vi "Generate Dashboard DVR.vi"(8 "Error In":errorcluster, 10 "Data":T1, 11 "Dashboard In":refnum<class "Dashboard.lvclass">) -> (0 "Error Out":errorcluster, 3 "Dashboard Out":refnum<class "Dashboard.lvclass">)   [LabVIEW 2019, in "Dashboard.lvclass"]
uses:
  Dashboard.lvclass
  Controls/Data.ctl
  Central Message Handler/Central Message Handler.lvclass
  <vilib>/Memosfet/myRIO-Neopixel/RT/Display/Display.lvclass
  Display Manager/Display Manager.lvclass
  Audio Analyzer/Audio Analyzer.lvclass
  Draw Frame/Draw Frame.lvclass
  Error Handling/Error Handling.lvclass
  Sequencer/Sequencer.lvclass
  <vilib>/Memosfet/OpenWeatherAPI/Open Weather Session/Open Weather Session.lvclass
  Public/Controls/FPGA Reference.ctl
  Controls/Processes.ctl
  Dashboard.lvclass/Dashboard.ctl
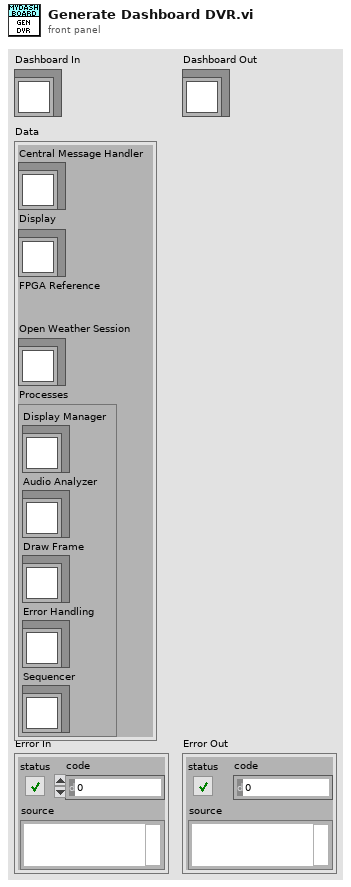
[diagram p1: front panel]
types:
  T1 = typedef "Dashboard.lvclass/Data.ctl" = cluster{"Central Message Handler":refnum<class "Central Message Handler.lvclass">, "Display":refnum<class "Display.lvclass">, "FPGA Reference":T2, "Open Weather Session":refnum<class "Open Weather Session.lvclass">, "Processes":T3}
  T2 = typedef "Dashboard.lvclass/FPGA Reference.ctl" = refnum<k20>
  T3 = typedef "Dashboard.lvclass/Processes.ctl" = cluster{"Display Manager":refnum<class "Display Manager.lvclass">, "Audio Analyzer":refnum<class "Audio Analyzer.lvclass">, "Draw Frame":refnum<class "Draw Frame.lvclass">, "Error Handling":refnum<class "Error Handling.lvclass">, "Sequencer":refnum<class "Sequencer.lvclass">}
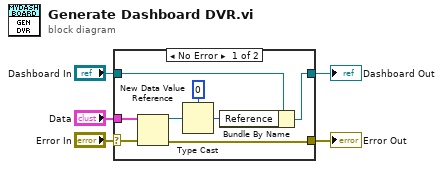
[diagram p0: block diagram]
diagram:
  n1 = case shown="No Error" "Error In" {
    selector: "Error In" -> [w13 w15]
    tunnel: "Dashboard In" -> [w10 w14]
    tunnel: [w7 w15] -> w4
    tunnel: [w8 w14] -> w2
    tunnel: "Data" -> [w6 _]
    frame No Error {
      n2 = New Data Value Reference(data value=w6, error in=w13) -> (data value reference=w11:refnum<data-value>, error out=w7:errorcluster)
      n3 = Type Cast(type=u64 0, x=w11) -> (*(type *) &x=w9:u64)
      n4 = Bundle By Name(cluster=w10, "Reference"=w9) -> (w8:refnum<class "Dashboard.lvclass">)
    }
    frame Error {
    }
  }
  "Error Out" <- w4
  "Dashboard Out" <- w2
